vi "Threshold VI.vi"(0 "Image In":T1, 1 "Green or Sat Range":cluster{"Lower value":i32, "Upper value":i32}={"Lower value"=131, "Upper value"=255} {"Lower value" scale=0.0..255.0; "Upper value" scale=0.0..255.0}, 2 "Red or Hue Range":cluster{"Lower value":i32, "Upper value":i32}={"Lower value"=3, "Upper value"=126} {"Lower value" scale=0.0..255.0; "Upper value" scale=0.0..255.0}, 3 "Image Dst":T1, 4 "Blue or Luma or Val or Inten Range":cluster{"Lower value":i32, "Upper value":i32}={"Lower value"=34, "Upper value"=255} {"Lower value" scale=0.0..255.0; "Upper value" scale=0.0..255.0}, 5 "error in":errorcluster) -> (6 "Image":T1(plugin-control), 8 "error out":errorcluster)   [LabVIEW 2020]
uses:
  <vilib>/vision/Image Controls.llb/IMAQ Image.ctl
  <vilib>/vision/NI_Vision_Development_Module.lvlib
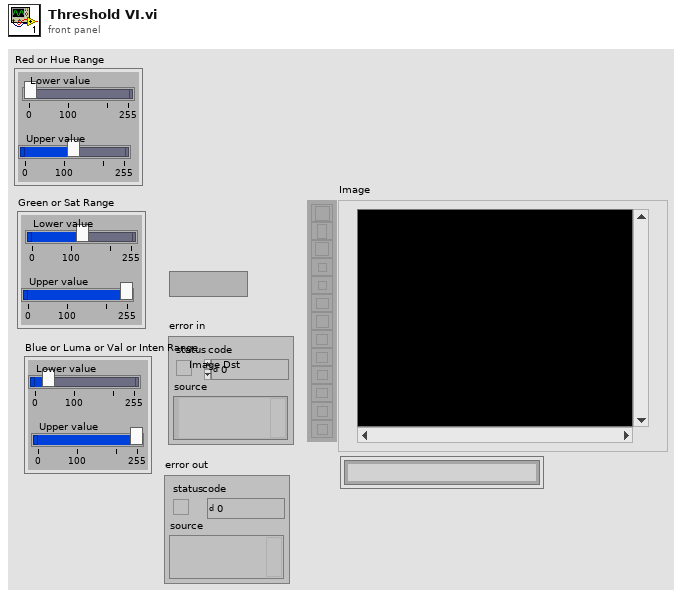
[diagram p1: front panel]
types:
  T1 = typedef "IMAQ Image.ctl" = refnum<image>
  T2 = typedef "Image Type" = u32
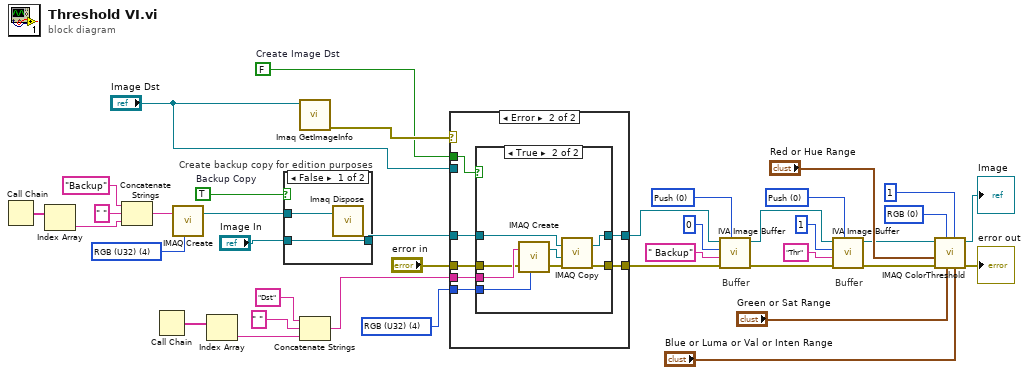
[diagram p0: block diagram]
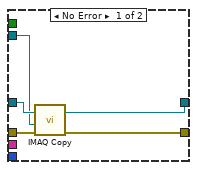
[diagram p2: hidden frame]
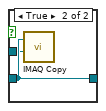
[diagram p4: hidden frame]
diagram:
  w7 = u16 0 items=["Push", "Pop", "Reset"] ("Function")
  w13 = u16 0 items=["RGB", "HSL", "HSV", "HSI"] ("Color Mode")
  w17 = u16 0 items=["Push", "Pop", "Reset"] ("Function")
  w20 = T2 4 items=["Grayscale (U8)", "Grayscale (I16)", "Grayscale (SGL)", "Complex (CSG)", "RGB (U32)", "HSL (U32)", "RGB (U64)", "Grayscale (U16)"] ("Image Dst Type")
  w21 = T2 4 items=["Grayscale (U8)", "Grayscale (I16)", "Grayscale (SGL)", "Complex (CSG)", "RGB (U32)", "HSL (U32)", "RGB (U64)", "Grayscale (U16)"] ("Image Type")
  w39 = TRUE  # Backup Copy
  w33 = FALSE  # Create Image Dst
  # "Buffer"
  # "Buffer"
  n1 = Call Chain() -> (call chain=w27:string[])
  n2 = Index Array(array=w27) -> (element=w26:string)  [unwired: 1 in]
  n3 = Concatenate Strings("Backup" ("Backup Image Name"), " ", w26) -> (w23:string)
  n4 = Call Chain() -> (call chain=w32:string[])
  n5 = call "IMAQ Create"("Image Name"=w23, "Image Type"=w21) -> ("New Image"=w22:T1)  [unwired: 2 in, 2 out]
  n6 = Index Array(array=w32) -> (element=w30:string)  [unwired: 1 in]
  n7 = case "Create backup copy for edition purposes" shown="False" w39 {
    tunnel: [w41 w43] -> w35
    tunnel: "Image In" -> [w41 w43]
    tunnel: w22 -> [w40 w42]
    frame False {
      n8 = call "Imaq Dispose"("Image"=w40) -> ()  [unwired: 2 in, 4 out]
    }
    frame True {
      n9 = call "IMAQ Copy"("Image Dst"=w42, "Image Src"=w43) -> ()  [unwired: 1 in, 5 out]
    }
  }
  n10 = call "Imaq GetImageInfo"("Image"="Image Dst") -> ("error out"=w37:errorcluster)  [unwired: 1 in, 9 out]
  n11 = Concatenate Strings("Dst" ("Image Dst Name"), " ", w30) -> (w28:string)
  n12 = case shown="Error" w37 {
    tunnel: [w48 w52] -> w19
    tunnel: [w47 w51] -> w18
    tunnel: w35 -> [w46 w53]
    tunnel: "error in" -> [w45 w49]
    tunnel: "Image Dst" -> [w44 _]
    tunnel: w28 -> [_ w55]
    tunnel: w20 -> [_ w54]
    tunnel: w33 -> [_ w50]
    frame No Error {
      n13 = call "IMAQ Copy"("error in (no error)"=w45, "Image Dst"=w44, "Image Src"=w46) -> ("error out"=w47:errorcluster, "Image Dst Out"=w48:T1)  [unwired: 3 out]
    }
    frame Error {
      n14 = case shown="True" w50 {
        tunnel: w55 -> [_ w65]
        tunnel: w54 -> [_ w64]
        tunnel: w53 -> [w57 w62]
        tunnel: [w57 w61] -> w52
        tunnel: [w56 w60] -> w51
        tunnel: w49 -> [w56 w58]
        frame False {
        }
        frame True {
          n15 = call "IMAQ Create"("Image Name"=w65, "Image Type"=w64, "error in (no error)"=w58) -> ("New Image"=w63:T1, "error out"=w59:errorcluster)  [unwired: 1 in, 1 out]
          n16 = call "IMAQ Copy"("error in (no error)"=w59, "Image Dst"=w63, "Image Src"=w62) -> ("error out"=w60:errorcluster, "Image Dst Out"=w61:T1)  [unwired: 3 out]
        }
      }
    }
  }
  n17 = call <vilib>:"IVA Image Buffer.vi"("Function"=w17, "error in (no error)"=w18, "Prefix"=" Backup", "Buffer #"=0, "Image In"=w19) -> ("error out"=w3:errorcluster, "Image Out"=w4:T1)  [unwired: 5 out]
  n18 = call <vilib>:"IVA Image Buffer.vi"("Function"=w7, "error in (no error)"=w3, "Prefix"="Thr", "Buffer #"=1, "Image In"=w4) -> ("error out"=w1:errorcluster, "Image Out"=w2:T1)  [unwired: 5 out]
  n19 = call "IMAQ ColorThreshold"("Blue or Luma or Val or Inten Range"="Blue or Luma or Val or Inten Range", "Replace Value"=1, "Green or Sat Range"="Green or Sat Range", "Color Mode"=w13, "error in (no error)"=w1, "Red or Hue Range"="Red or Hue Range", "Image Src"=w2) -> ("error out"=→"error out":errorcluster, "Image Dst Out"=→"Image":T1)  [unwired: 1 in, 2 out]
